vi "Perform Action.vi"(8 "error in":errorcluster, 9 "Input":variant, 10 "Task.Point Ident":string, 11 "MSS Target Actor in":refnum<class "MSS Target Actor.lvclass">) -> (0 "error out":errorcluster, 1 "Output":variant, 3 "MSS Target Actor out":refnum<class "MSS Target Actor.lvclass">)   [LabVIEW 2023, in "MSS Target Actor.lvlib" / "MSS Target Actor.lvclass"]
uses:
  MSS Target Actor.lvclass
  MSS Target Actor.lvclass/MSS Target Actor.ctl
  MSS/MSS.lvclass
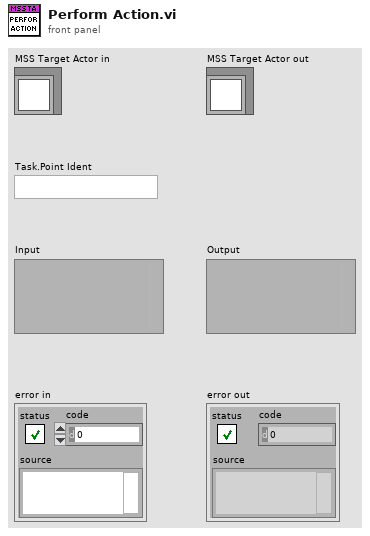
[diagram p1: front panel]
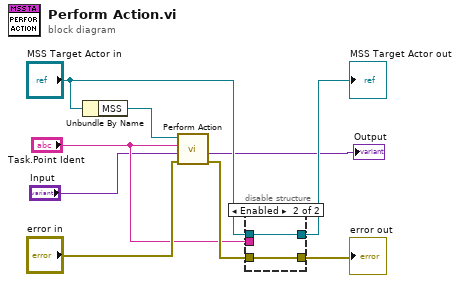
[diagram p0: block diagram]
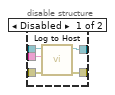
[diagram p2: hidden frame]
diagram:
  n1 = Unbundle By Name("MSS Target Actor in") -> ("MSS"=w9:refnum<class "MSS.lvclass">)
  n2 = call "Perform Action.vi"("error in"="error in", "Input"="Input", "Point Ident"="Task.Point Ident", "MSS in"=w9) -> ("error out"=w7:errorcluster, "Output"=→"Output":variant)  [unwired: 4 in, 2 out]
  n3 = disable-structure shown="Enabled" {
    disable-tunnel: w7 -> [w14 w15]
    disable-tunnel: [w13 w15] -> w6
    disable-tunnel: "MSS Target Actor in" -> [w12 w16]
    disable-tunnel: [w11 w16] -> w4
    disable-tunnel: "Task.Point Ident" -> [w10 _]
    frame Disabled {
      n4 = call "Log to Host.vi"("error in"=w14, "Detail"=w10, "MSS Target Actor in"=w12) -> ("error out"=w13:errorcluster, "MSS Target Actor out"=w11:refnum<class "MSS Target Actor.lvclass">)  [unwired: 7 in]
    }
    frame Enabled {
    }
  }
  "error out" <- w6
  "MSS Target Actor out" <- w4
